vi "read-autofocus-file.vi"   [LabVIEW 2014]
uses:
  save-autofocus-global.vi
  <vilib>/Utility/config.llb/Read Key (Boolean).vi
  TIRF Lock/autofocus-globals.vi
  <vilib>/Utility/config.llb/Read Key (Double).vi
  <vilib>/Utility/config.llb/Read Key (I32).vi
  <vilib>/Utility/config.llb/NI_LVConfig.lvlib
types:
  T1 = enum32{"Invalid", "Standard", "Closed", "Hidden", "Minimized", "Maximized"}
  T2 = typedef "NI_LVConfig.lvlib/Config Data RefNum.ctl" = refnum<k1>
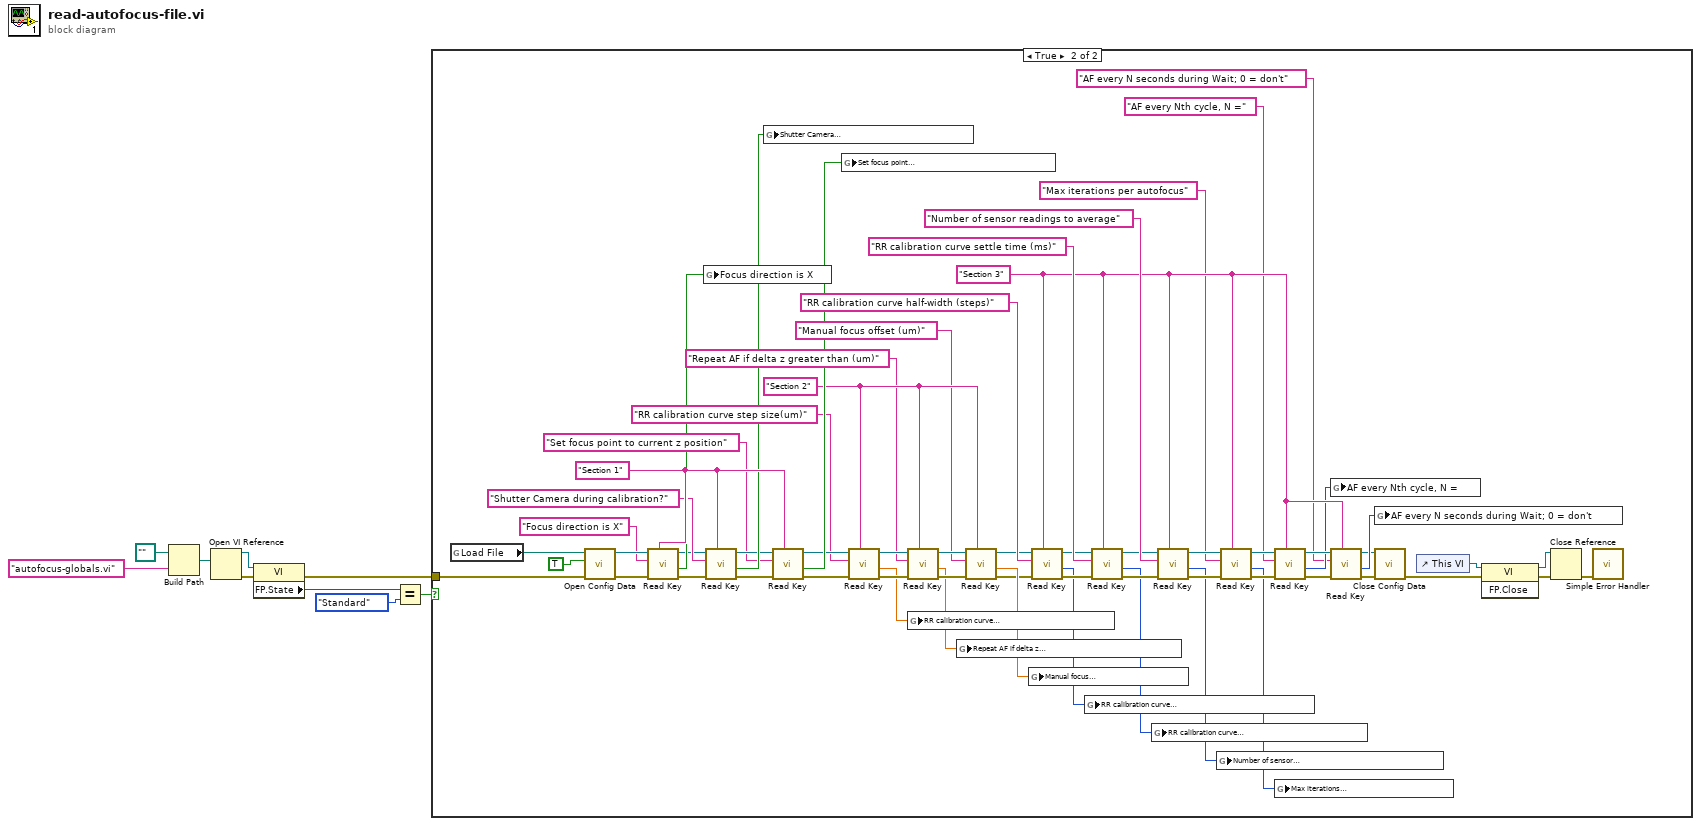
[diagram p0: block diagram]
diagram:
  n1 = Build Path(base path=path "", name or relative path="autofocus-globals.vi") -> (appended path=w8:path)
  n2 = Open VI Reference(vi path=w8) -> (vi reference=w7:refnum<vi>, error out=w6:errorcluster)  [unwired: 1 in, 4 out]
  n3 = property class="VI"(reference=w7, error in=w6) -> (error out=w2:errorcluster, "FP.State"=w3:T1)  [unwired: 1 out]
  n4 = Equal?(x=w3, y=T1."Standard") -> (x = y?=w1:bool)
  n5 = case shown="True" w1 {
    tunnel: w2 -> [_ w68]
    frame False {
    }
    frame True {
      w23 = "Section 3"
      w48 = "Section 2"
      w63 = "Section 1"
      n6 = global read "save-autofocus-global.vi" "Load File"() -> (w70:path)
      n7 = call <vilib>:"Open Config Data.vi"("error in (no error)"=w68, "create file if necessary (T)"=TRUE, "configuration file path"=w70) -> ("error out"=w67:errorcluster, "refnum"=w66:T2)  [unwired: 6 in, 1 out]
      n8 = call-poly <vilib>:"Read Key.vi"("section"=w63, "error in (no error)"=w67, "key"="Focus direction is X", "refnum"=w66) -> ("error out"=w65:errorcluster, "value"=w62:bool, "refnum out"=w57:T2)  [unwired: 1 in, 4 out]
      n9 = global write "autofocus-globals.vi" "Focus direction is X"(w62) -> ()
      n10 = call-poly <vilib>:"Read Key.vi"("section"=w63, "error in (no error)"=w65, "key"="Shutter Camera during calibration?", "refnum"=w57) -> ("error out"=w64:errorcluster, "value"=w61:bool, "refnum out"=w56:T2)  [unwired: 1 in, 4 out]
      n11 = global write "autofocus-globals.vi" "Shutter Camera\nduring calibration?"(w61) -> ()
      n12 = call-poly <vilib>:"Read Key.vi"("section"=w63, "error in (no error)"=w64, "key"="Set focus point to current z position", "refnum"=w56) -> ("error out"=w54:errorcluster, "value"=w60:bool, "refnum out"=w53:T2)  [unwired: 1 in, 4 out]
      n13 = global write "autofocus-globals.vi" "Set focus point\nto current z position"(w60) -> ()
      n14 = call-poly <vilib>:"Read Key.vi"("section"=w48, "error in (no error)"=w54, "key"="RR calibration curve step size(um)", "refnum"=w53) -> ("error out"=w52:errorcluster, "value"=w44:dbl, "refnum out"=w51:T2)  [unwired: 1 in, 4 out]
      n15 = call-poly <vilib>:"Read Key.vi"("section"=w48, "error in (no error)"=w52, "key"="Repeat AF if delta z greater than (um)", "refnum"=w51) -> ("error out"=w50:errorcluster, "value"=w42:dbl, "refnum out"=w49:T2)  [unwired: 1 in, 4 out]
      n16 = global write "autofocus-globals.vi" "RR calibration curve\nstep size (um)"(w44) -> ()
      n17 = global write "autofocus-globals.vi" "Repeat AF if delta z \ngreater than (um)"(w42) -> ()
      n18 = call-poly <vilib>:"Read Key.vi"("section"=w48, "error in (no error)"=w50, "key"="Manual focus offset (um)", "refnum"=w49) -> ("error out"=w41:errorcluster, "value"=w47:dbl, "refnum out"=w29:T2)  [unwired: 1 in, 4 out]
      n19 = global write "autofocus-globals.vi" "Manual focus\noffset (um)"(w47) -> ()
      n20 = call-poly <vilib>:"Read Key.vi"("section"=w23, "error in (no error)"=w41, "key"="RR calibration curve half-width (steps)", "refnum"=w29) -> ("error out"=w40:errorcluster, "value"=w34:i32, "refnum out"=w28:T2)  [unwired: 4 in, 1 out]
      n21 = global write "autofocus-globals.vi" "RR calibration curve\nhalf-width  (steps)"(w34) -> ()
      n22 = call-poly <vilib>:"Read Key.vi"("section"=w23, "error in (no error)"=w40, "key"="RR calibration curve settle time (ms)", "refnum"=w28) -> ("error out"=w39:errorcluster, "value"=w33:i32, "refnum out"=w27:T2)  [unwired: 4 in, 1 out]
      n23 = global write "autofocus-globals.vi" "RR calibration curve\nsettle time (ms)"(w33) -> ()
      n24 = call-poly <vilib>:"Read Key.vi"("section"=w23, "error in (no error)"=w39, "key"="Number of sensor readings to average", "refnum"=w27) -> ("error out"=w38:errorcluster, "value"=w30:i32, "refnum out"=w26:T2)  [unwired: 4 in, 1 out]
      n25 = global write "autofocus-globals.vi" "Number of sensor\nreadings to average"(w30) -> ()
      n26 = call-poly <vilib>:"Read Key.vi"("section"=w23, "error in (no error)"=w38, "key"="Max iterations per autofocus", "refnum"=w26) -> ("error out"=w37:errorcluster, "value"=w22:i32, "refnum out"=w25:T2)  [unwired: 4 in, 1 out]
      n27 = call-poly <vilib>:"Read Key.vi"("section"=w23, "error in (no error)"=w37, "key"="AF every Nth cycle, N =", "refnum"=w25) -> ("error out"=w36:errorcluster, "value"=w20:i32, "refnum out"=w24:T2)  [unwired: 4 in, 1 out]
      n28 = global write "autofocus-globals.vi" "Max iterations \nper autofocus"(w22) -> ()
      n29 = global write "autofocus-globals.vi" "AF every Nth cycle, N ="(w20) -> ()
      n30 = call-poly <vilib>:"Read Key.vi"("section"=w23, "error in (no error)"=w36, "key"="AF every N seconds during Wait; 0 = don't", "refnum"=w24) -> ("error out"=w16:errorcluster, "value"=w19:i32, "refnum out"=w15:T2)  [unwired: 4 in, 1 out]
      n31 = global write "autofocus-globals.vi" "AF every N seconds during Wait; 0 = don't"(w19) -> ()
      n32 = call <vilib>:"Close Config Data.vi"("error in (no error)"=w16, "refnum"=w15) -> ("error out"=w10:errorcluster)  [unwired: 1 in, 8 out]
      n33 = control-ref of="This VI"() -> (w14:refnum<vi>)
      n34 = invoke class="VI" method="FP.Close"(reference=w14, error in=w10) -> (reference out=w12:refnum<vi>, error out=w11:errorcluster)  [unwired: 1 in, 1 out]
      n35 = Close Reference(reference=w12, error in (no error)=w11) -> (error out=w13:errorcluster)
      n36 = call <vilib>:"Simple Error Handler.vi"("error in (no error)"=w13) -> ()  [unwired: 4 in, 5 out]
    }
  }
